vi "Electronique.vi"() -> ()   [LabVIEW 2018]
panel:
  in  "Numeric":dbl
  out "Boolean 6":bool
  out "Boolean 5":bool
  out "Boolean 4":bool
  out "Boolean 3":bool
  out "Boolean 2":bool
  out "Led":bool
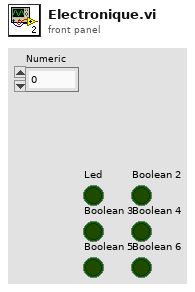
[diagram p1: front panel]
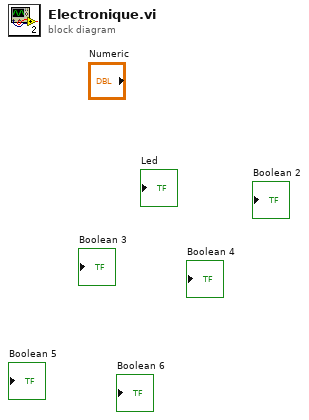
[diagram p0: block diagram]
diagram:
